vi "G#Object_RegisterExternalCreateProcessCallers.vi"(1 "Action":T1(ring), 5 "error in (no error)":errorcluster) -> (15 "StopExternalCreate?":bool, 19 "error out":errorcluster)   [LabVIEW 2017, in "G#Object.lvclass"]
doc: "Registers or deregister top-level callesrs."
uses:
  G#Object.lvclass
  <vilib>/Utility/error.llb/Error Cluster From Error Code.vi
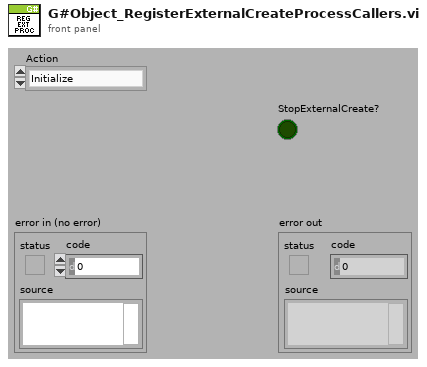
[diagram p1: front panel]
types:
  T1 = enum16{"Initialize", "Register", "Unregister", "Clear"}
  T2 = enum32{"Bad", "Idle", "Run top level", "Running"}
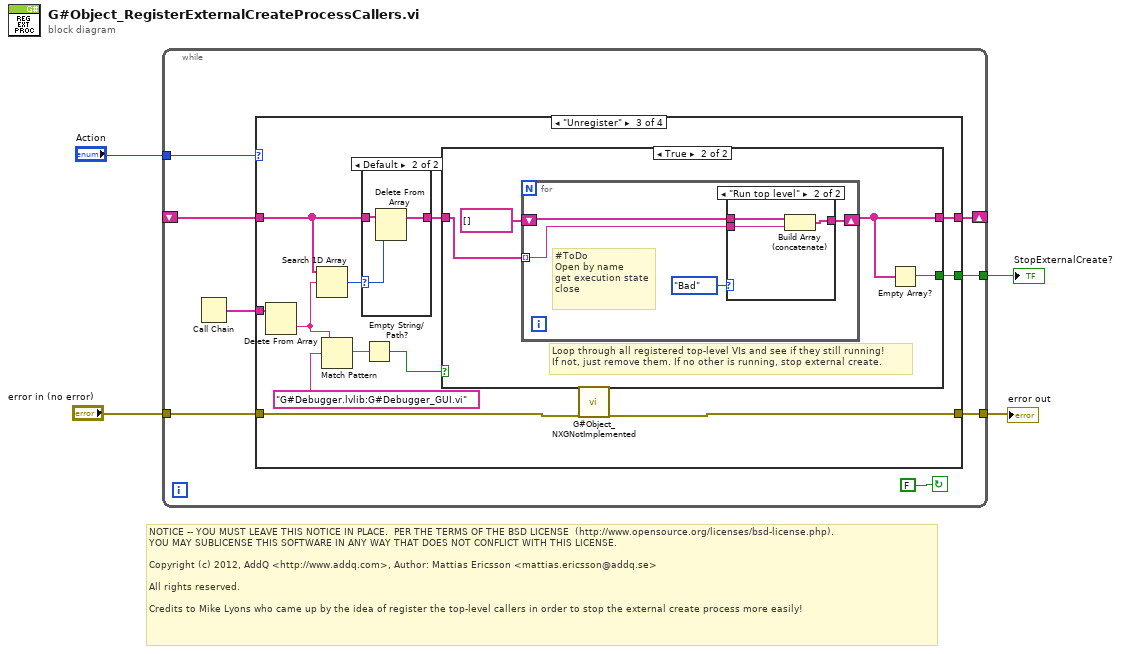
[diagram p0: block diagram]
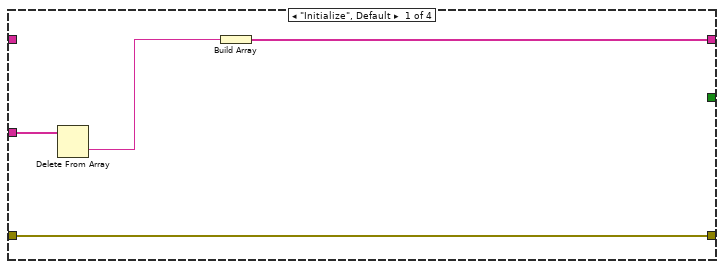
[diagram p2: hidden frame]
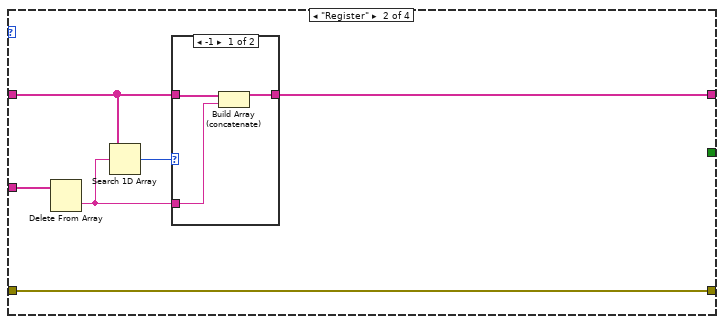
[diagram p3: hidden frame]
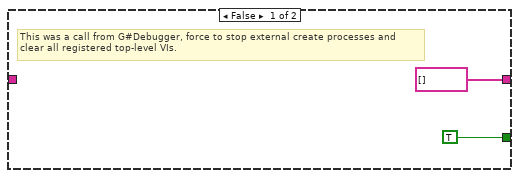
[diagram p5: hidden frame]
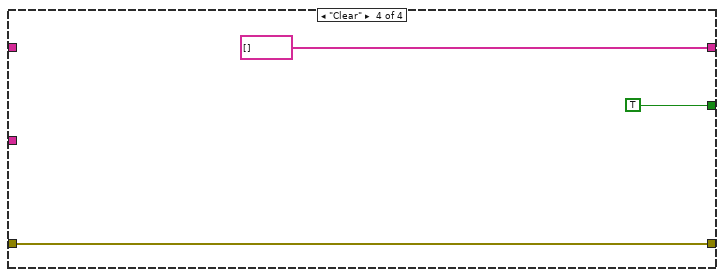
[diagram p8: hidden frame]
diagram:
  # "NOTICE -- YOU MUST LEAVE THIS NOTICE IN PLACE.  PER THE TERMS OF THE BSD LICENSE  (http://www.opensource.org/licenses/bsd-license.php).\nYOU MAY SUBLICENSE THIS SOFTWARE IN ANY WAY THAT DOES NOT CONFLICT WITH THIS LICENSE.\n\nCopyright (c) 2012, AddQ <http://www.addq.com>, Author: Mattias Ericsson <mattias.ericsson@addq.se>\n\nAll rights reserved.\n\nCredits to Mike Lyons who came up by the idea of register the top-level callers in order to stop the external create process more easily!"
  n1 = while {
    tunnel: "error in (no error)" -> [w11]
    tunnel: "Action" -> [w12]
    shift-right: [w8] -> _
    shift-left: _ -> [w6]
    tunnel: [w7] -> w2
    tunnel: [w5] -> w1
    stop <- FALSE continue-if-true
    n2 = Call Chain() -> (call chain=w9:string[])
    n3 = case shown="\"Unregister\"" w12 {
      tunnel: w11 -> [w13 w17 w28 w58]
      tunnel: w9 -> [w16 w22 w38 _]
      tunnel: [w15 w19 w33 string[] []] -> w8
      tunnel: [w13 w17 w27 w58] -> w7
      tunnel: w6 -> [_ w20 w36 _]
      tunnel: [_ _ w34 TRUE] -> w5
      frame "Initialize", Default {
        n4 = Delete From Array(array=w16) -> (deleted portion=w14:string)  [unwired: 2 in, 1 out]
        n5 = Build Array(w14) -> (w15:string[])
      }
      frame "Register" {
        n6 = Delete From Array(array=w22) -> (deleted portion=w18:string)  [unwired: 2 in, 1 out]
        n7 = Search 1D Array(1D array=w20, element=w18) -> (index of element=w21:i32)  [unwired: 1 in]
        n8 = case shown="-1" w21 {
          tunnel: w20 -> [w25 w26]
          tunnel: [w23 w26] -> w19
          tunnel: w18 -> [w24 _]
          frame -1 {
            n9 = Build Array (concatenate)(w25, w24) -> (w23:string[])
          }
          frame Default {
          }
        }
      }
      frame "Unregister" {
        n10 = Delete From Array(array=w38) -> (deleted portion=w32:string)  [unwired: 2 in, 1 out]
        n11 = Search 1D Array(1D array=w36, element=w32) -> (index of element=w37:i32)  [unwired: 1 in]
        n12 = Match Pattern(string=w32, regular expression="G#Debugger.lvlib:G#Debugger_GUI.vi") -> (match substring=w30:string)  [unwired: 1 in, 3 out]
        n13 = case shown="Default" w37 {
          selector: w37 -> [_ w54]
          tunnel: w36 -> [w53 w56]
          tunnel: [w53 w55] -> w35
          frame -1 {
          }
          frame Default {
            n14 = Delete From Array(array=w56, index=w54) -> (array with subset deleted=w55:string[])  [unwired: 1 in, 1 out]
          }
        }
        n15 = Empty String/Path?(string/path=w30) -> (empty?=w29:bool)
        n16 = case shown="True" w29 {
          tunnel: w35 -> [_ w44]
          tunnel: [TRUE w42] -> w34
          tunnel: [string[] [] w41] -> w33
          frame False {
            # "This was a call from G#Debugger, force to stop external create processes and\nclear all registered top-level VIs."
          }
          frame True {
            # "Loop through all registered top-level VIs and see if they still running!\nIf not, just remove them. If no other is running, stop external create."
            n17 = for {
              tunnel: w44 -> [w48] mode=indexing
              shift-right: [w46] -> w41
              shift-left: string[] [] -> [w47]
              # "#ToDo\nOpen by name\nget execution state\nclose"
              n18 = case shown="\"Run top level\"" T2."Bad" ("Exec.State") {
                tunnel: w48 -> [_ w51]
                tunnel: w47 -> [w49 w52]
                tunnel: [w49 w50] -> w46
                frame Default {
                }
                frame "Run top level" {
                  n19 = Build Array (concatenate)(w52, w51) -> (w50:string[])
                }
              }
            }
            n20 = Empty Array?(array=w41) -> (empty?=w42:bool)
          }
        }
        n21 = call "G#Object_NXGNotImplemented.vi"("error in"=w28) -> ("error out"=w27:errorcluster)  [unwired: 18 in]
      }
      frame "Clear" {
      }
    }
  }
  "error out" <- w2
  "StopExternalCreate?" <- w1
